vi "GenGradient.vi"(5 "Color 2":u32(colorbox)=16860, 6 "Reset":bool, 7 "Color 1":u32(colorbox)=16711680, 10 "Sine Rate":i32, 11 "NumLeds":i32) -> (3 "LED Array":u32[](array[numeric]))   [LabVIEW 2018, in "ArduinoSerialBling.lvlib"]
uses:
  ArduinoSerialBling.lvlib
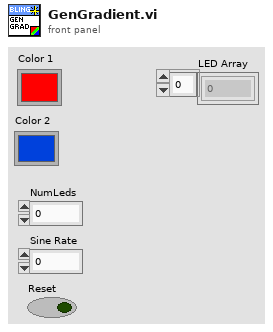
[diagram p1: front panel]
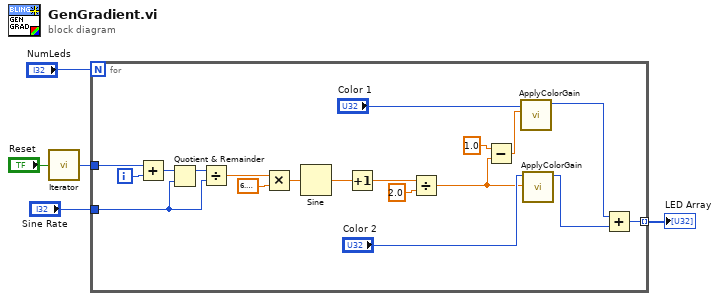
[diagram p0: block diagram]
diagram:
  n1 = call "Iterator.vi"("Reset"="Reset") -> ("i"=w2:i32)
  n2 = for {
    N: "NumLeds" -> [_]
    tunnel: [w10] -> w5 mode=indexing
    tunnel: "Sine Rate" -> [w13]
    tunnel: w2 -> [w12]
    i -> [w11]
    n3 = Add(x=w12, y=w11) -> (x+y=w14:i32)
    n4 = Quotient & Remainder(x=w14, y=w13) -> (x-y*floor(x/y)=w16:i32)  [unwired: 1 out]
    n5 = Divide(x=w16, y=w13) -> (x/y=w17:dbl)
    n6 = Multiply(x=w17, y=6.283185307179586) -> (x*y=w18:dbl)
    n7 = Sine(x=w18) -> (sin(x)=w19:dbl)
    n8 = Increment(x=w19) -> (x+1=w20:dbl)
    n9 = Divide(x=w20, y=2.0) -> (x/y=w6:dbl)
    n10 = Subtract(x=1.0, y=w6) -> (x-y=w22:dbl)
    n11 = call "ApplyColorGain.vi"("Gain"=w22, "Color In"="Color 1") -> ("Color Out"=w9:u32)  [unwired: 9 in]
    n12 = call "ApplyColorGain.vi"("Gain"=w6, "Color In"="Color 2") -> ("Color Out"=w8:u32)  [unwired: 9 in]
    n13 = Add(x=w9, y=w8) -> (x+y=w10:u32)
  }
  "LED Array" <- w5
